vi "Reconnection_Update_Of_FGV.vi"(11 "user":i32) -> ()   [LabVIEW 2020]
panel:
  out "user":i32
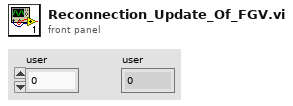
[diagram p1: front panel]
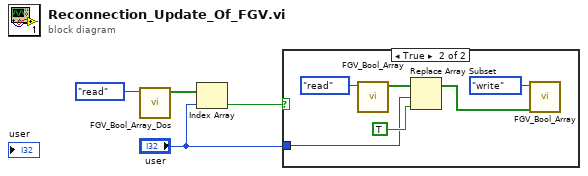
[diagram p0: block diagram]
diagram:
  n1 = call "FGV_Bool_Array_Dos.vi"("Enum"=enum16{"read", "write"}."read" ("operation (0:open)")) -> ("Array Out"=w3:bool[])  [unwired: 10 in]
  n2 = Index Array(array=w3, index="user") -> (element=w2:bool)
  n3 = case shown="True" w2 {
    tunnel: "user" -> [_ w5]
    frame False {
    }
    frame True {
      n4 = call "FGV_Bool_Array.vi"("Enum"=enum16{"read", "write"}."read") -> ("Array Out"=w10:bool[])  [unwired: 10 in]
      n5 = Replace Array Subset(array=w10, new element=TRUE, index=w5) -> (w6:bool[])
      n6 = call "FGV_Bool_Array.vi"("Array In"=w6, "Enum"=enum16{"read", "write"}."write") -> ()  [unwired: 9 in, 1 out]
    }
  }
